vi "Prediction.vi"(8 "error in (no error)":errorcluster, 11 "Measurement in":refnum<class "Measurement.lvclass">) -> (0 "error out":errorcluster, 2 "Numeric":i64, 3 "Measurement out":refnum<class "Measurement.lvclass">)   [LabVIEW 2020, in "Measurement.lvclass"]
uses:
  Measurement.lvclass
  Measurement.lvclass/Measurement.ctl
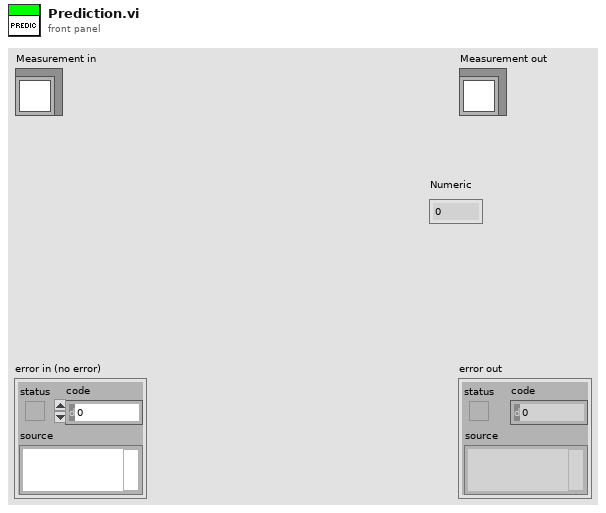
[diagram p1: front panel]
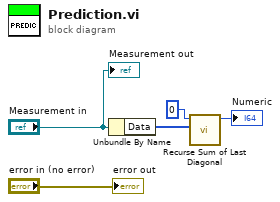
[diagram p0: block diagram]
diagram:
  n1 = Unbundle By Name("Measurement in") -> ("Data"=w3:i64[])
  n2 = call "Recurse Sum of Last Diagonal.vi"("Data"=w3, "Numeric in"=i64 0 ("Numeric")) -> ("Numeric out"=→"Numeric":i64)  [unwired: 9 in]
  "error out" <- "error in (no error)"
  "Measurement out" <- "Measurement in"
